vi "Inficon - Connect.vi"(8 "Error In":errorcluster, 11 "COM in":refnum<visa-resource-name>) -> (0 "Error Out":errorcluster, 3 "COM out":refnum<visa-resource-name>)   [LabVIEW 2014]
uses:
  <vilib>/Instr/_visa.llb/VISA Configure Serial Port (Instr).vi
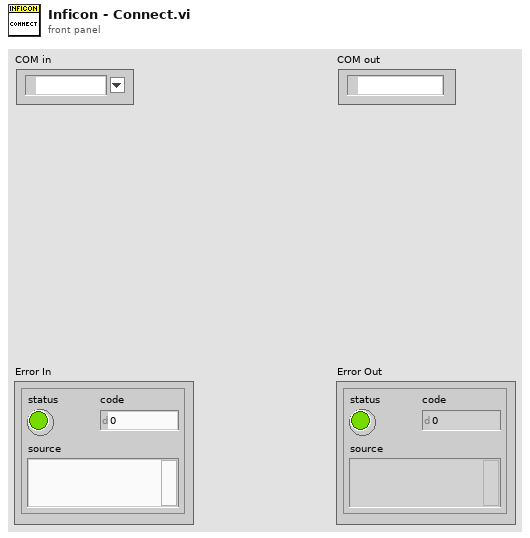
[diagram p1: front panel]
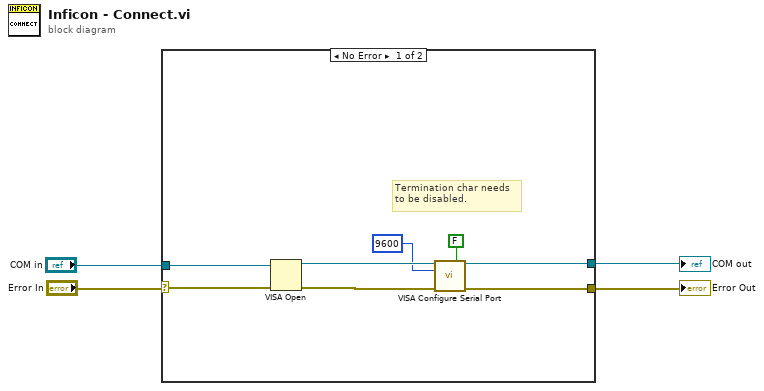
[diagram p0: block diagram]
diagram:
  n1 = case shown="No Error" "Error In" {
    selector: "Error In" -> [w12 w13]
    tunnel: [w10 w13] -> w3
    tunnel: "COM in" -> [w9 w14]
    tunnel: [w7 w14] -> w1
    frame No Error {
      # "Termination char needs\nto be disabled."
      n2 = VISA Open(error in (no error)=w12, VISA resource name=w9) -> (VISA resource name=w8:refnum<visa-resource-name>, error out=w11:errorcluster)  [unwired: 3 in]
      n3 = call-poly "VISA Configure Serial Port"("VISA resource name"=w8, "Enable Termination\nChar (T)"=FALSE ("Enable Termination\nChar (T)"), "baud rate (9600)"=u32 9600, "error in (no error)"=w11) -> ("VISA resource name out"=w7:refnum<visa-resource-name>, "error out"=w10:errorcluster)  [unwired: 10 in]
    }
    frame Error {
    }
  }
  "Error Out" <- w3
  "COM out" <- w1
